vi "Untitled 2.vi"() -> ()   [LabVIEW 2019]
uses:
  <vilib>/userDefined/High Color/IMAQdx.ctl
  <vilib>/vision/driver/NI_Vision_Acquisition_Software.lvlib
  <vilib>/vision/NI_Vision_Development_Module.lvlib
panel:
  in  "stop":bool
  out "Read String":string
  out "Image":T1(plugin-control)
  in  "Rectangle":T2 {"Rotation" min=-90.0 max=90.0 step=1.0 format="%.2f"; "Left" scale=0.0..1024.0; "Right" scale=0.0..1024.0}
  in  "File Path":path
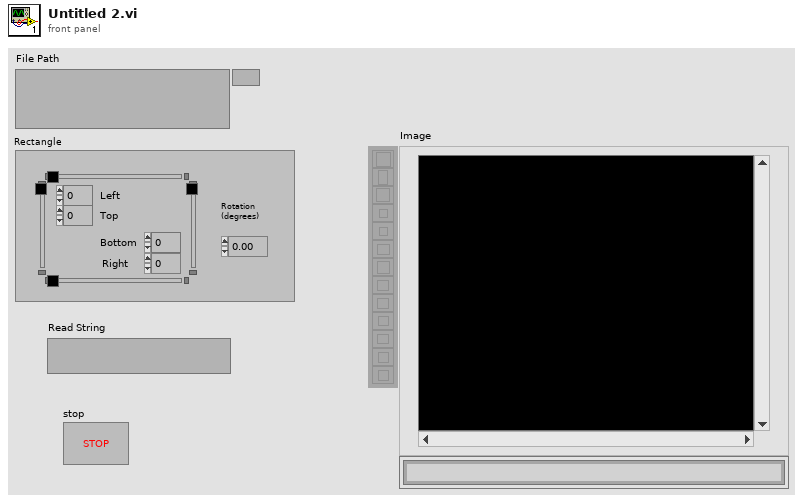
[diagram p1: front panel]
types:
  T1 = typedef "IMAQ Image.ctl" = refnum<image>
  T2 = typedef "IMAQ Rectangle" = cluster{"Left":i32, "Top":i32, "Right":i32, "Bottom":i32, "Rotation":dbl}
  T3 = typedef "IMAQdx.ctl" = refnum<k21>
  T4 = typedef "IMAQ OCR Session.ctl" = refnum<k1>
  T5 = typedef "ROI Descriptor" = cluster{"Global Rectangle":i32[], "Contours":cluster{"ID":enum32{"External", "Internal"}, "Type":u32, "Coordinates":i32[]}[]}
  T6 = cluster{"Global Rectangle":i32[], "Contours":cluster{"ID":enum32{"External", "Internal"}, "Type":u32, "Coordinates":i32[]}[]}
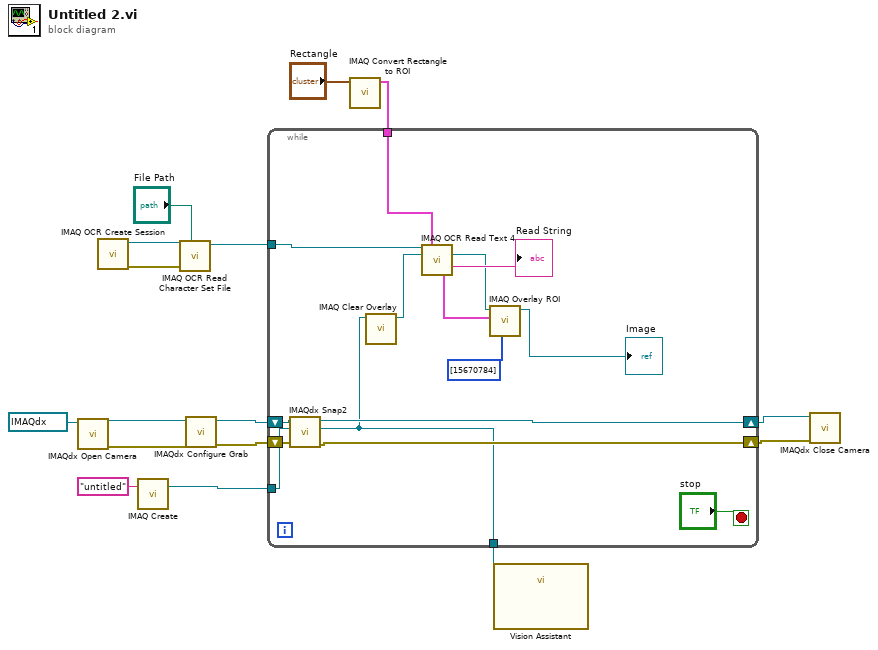
[diagram p0: block diagram]
diagram:
  n1 = call <vilib>:"IMAQdx Open Camera.vi"("Session In"=T3 "cam5") -> ("error out"=w12:errorcluster, "Session Out"=w15:T3)  [unwired: 9 in]
  n2 = call "IMAQ OCR Create Session"() -> ("error out"=w5:errorcluster, "IMAQ OCR Session"=w6:T4)  [unwired: 10 in]
  n3 = call "IMAQ Create"("Image Name"="untitled") -> ("New Image"=w9:T1)  [unwired: 4 in, 1 out]
  n4 = call "IMAQ OCR Read Character Set File"("File Path"="File Path", "error in (no error)"=w5, "IMAQ OCR Session"=w6) -> ("IMAQ OCR Session (dup)"=w3:T4)  [unwired: 6 in, 2 out]
  n5 = call <vilib>:"IMAQdx Configure Grab.vi"("error in"=w12, "Session In"=w15) -> ("error out"=w11:errorcluster, "Session Out"=w14:T3)  [unwired: 8 in]
  n6 = call "IMAQ Convert Rectangle to ROI"("Rectangle"="Rectangle") -> ("ROI Descriptor"=w2:T5)  [unwired: 8 in, 1 out]
  n7 = while {
    tunnel: w9 -> [w27]
    shift-right: [w30] -> w13
    shift-left: w14 -> [w31]
    shift-right: [w28] -> w10
    shift-left: w11 -> [w29]
    tunnel: [w19] -> w7
    tunnel: w3 -> [w17]
    tunnel: w2 -> [w26]
    stop <- "stop" stop-if-true
    n8 = call <vilib>:"IMAQdx Snap2.vi"("error in"=w29, "Image In"=w27, "Session In"=w31) -> ("error out"=w28:errorcluster, "Image Out"=w19:T1, "Session Out"=w30:T3)  [unwired: 6 in]
    n9 = call "IMAQ Clear Overlay"("Image"=w19) -> ("Image Out"=w18:T1)  [unwired: 9 in, 1 out]
    n10 = call "IMAQ OCR Read Text 4"("IMAQ OCR Session"=w17, "ROI Descriptor"=w26, "Image"=w18) -> ("Image (dup)"=w22:T1, "Read String"=→"Read String":string, "ROI Bounding Characters"=w23:T6)  [unwired: 6 in, 4 out]
    n11 = call "IMAQ Overlay ROI"("Colors (Green)"=u32[] [15670784], "ROI Descriptor"=w23, "Image"=w22) -> ("Image Out"=→"Image":T1)  [unwired: 7 in, 1 out]
  }
  n12 = call "Vision Assistant"("Image In"=w7) -> ()  [unwired: 25 in, 2 out]
  n13 = call <vilib>:"IMAQdx Close Camera.vi"("error in"=w10, "Session In"=w13) -> ()  [unwired: 9 in, 1 out]
